vi "detOf3X3.vi"(1 "3x3 matrix":dbl[][](array[numeric])) -> (0 "Determinant":dbl)   [LabVIEW 2015]
doc: "3x3 array -- It's a 3x3 aray type.\nDeterminant -- The determinant of the 3x3 matrix."
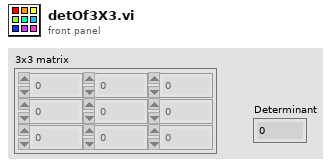
[diagram p1: front panel]
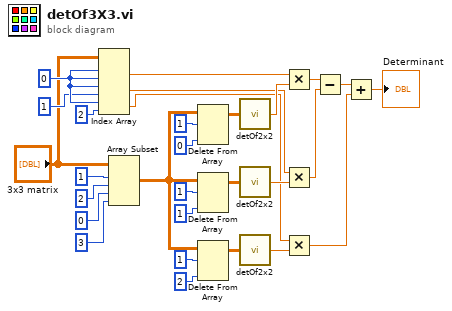
[diagram p0: block diagram]
diagram:
  w29 = 0 ("index (row)")
  n1 = Index Array(array="3x3 matrix", index (row) #1=w29, index (col) #1=w29, index (row) #2=w29, index (col) #2=1 ("disabled index (col)"), index (row) #3=w29, index (col) #3=2 ("disabled index (col)")) -> (element #1=w13:dbl, element #2=w11:dbl, element #3=w8:dbl)
  n2 = Array Subset(array="3x3 matrix", index (row)=1 ("index"), length (row)=2 ("length"), index (col)=0 ("index"), length (col)=3 ("length")) -> (w15:dbl[][])
  n3 = Delete From Array(array=w15, length=1, index (col)=0 ("disabled index (col)")) -> (array with subset deleted=w14:dbl[][])  [unwired: 1 in, 1 out]
  n4 = Delete From Array(array=w15, length=1, index (col)=1 ("disabled index (col)")) -> (array with subset deleted=w10:dbl[][])  [unwired: 1 in, 1 out]
  n5 = Delete From Array(array=w15, length=1, index (col)=2 ("disabled index (col)")) -> (array with subset deleted=w7:dbl[][])  [unwired: 1 in, 1 out]
  n6 = call "detOf2x2.vi"("2x2Matrix"=w14) -> ("Determinant"=w12:dbl)
  n7 = call "detOf2x2.vi"("2x2Matrix"=w10) -> ("Determinant"=w9:dbl)
  n8 = call "detOf2x2.vi"("2x2Matrix"=w7) -> ("Determinant"=w6:dbl)
  n9 = Multiply(x=w13, y=w12) -> (x*y=w5:dbl)
  n10 = Multiply(x=w11, y=w9) -> (x*y=w4:dbl)
  n11 = Multiply(x=w8, y=w6) -> (x*y=w2:dbl)
  n12 = Subtract(x=w5, y=w4) -> (x-y=w3:dbl)
  n13 = Add(x=w3, y=w2) -> (x+y=→"Determinant":dbl)
